vi "Create Test Configuration.vi"() -> (0 "error out":errorcluster, 1 "Channel Names":string[](array[string]), 2 "Lines":T1[](array[typedef]), 3 "Module Configuration":refnum<class "Sequencer Module configuration.lvclass">, 4 "Channels":refnum<class "TBM channel.lvclass">[](array[class]), 5 "instance identifier":string)   [LabVIEW 2015, in "Sequencer Module tests.lvlib"]
doc: "This VI creates a standard test configuration for other unit tests. It currently creates and adds one line with every datatype to the module configuration."
uses:
  Sequencer Module tests.lvlib
  module/configuration/Sequencer Module configuration.lvclass
  <vilib>/NI/Tag Bus Module Framework/channel/TBM channel.lvclass
  module/configuration/Line.ctl
  classes/Sequence/Config/Sequence Config.lvclass
  classes/Result Processor/Config/ResultProcessor Config.lvclass
  classes/Report/On-The-Fly/Config/OnTheFlyReport Config.lvclass
  classes/Report Formatters/csv/Config/csv-formatter Config.lvclass
  <vilib>/NI/Tag Bus/tag/tag descriptor.lvclass/tag descriptor.ctl
  <vilib>/NI/Configuration Framework/serializable configuration/NISE_CEF_serializable configuration.lvclass
  <vilib>/NI/Tag Bus/tag/tag descriptor.lvclass
panel:
  out "Line Names":string[](array[string])
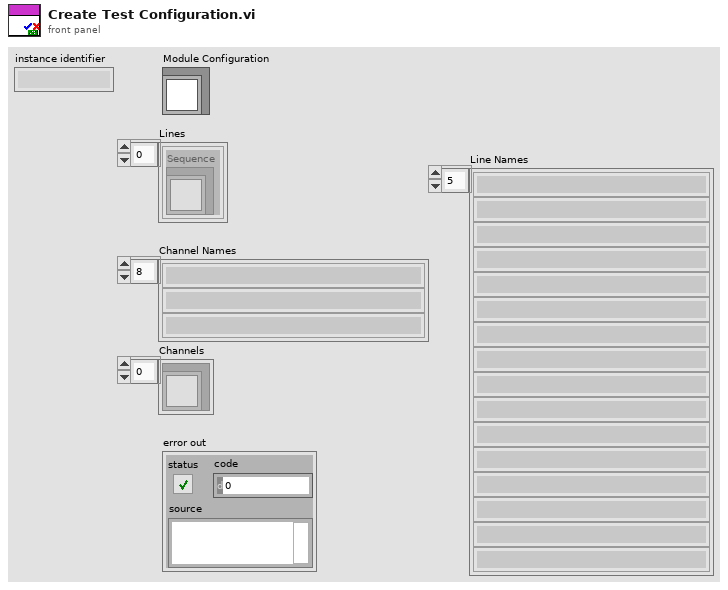
[diagram p1: front panel]
types:
  T1 = typedef "Sequencer Module configuration.lvclass/Line.ctl" = cluster{"Sequence":refnum<class "Sequence Config.lvclass">}
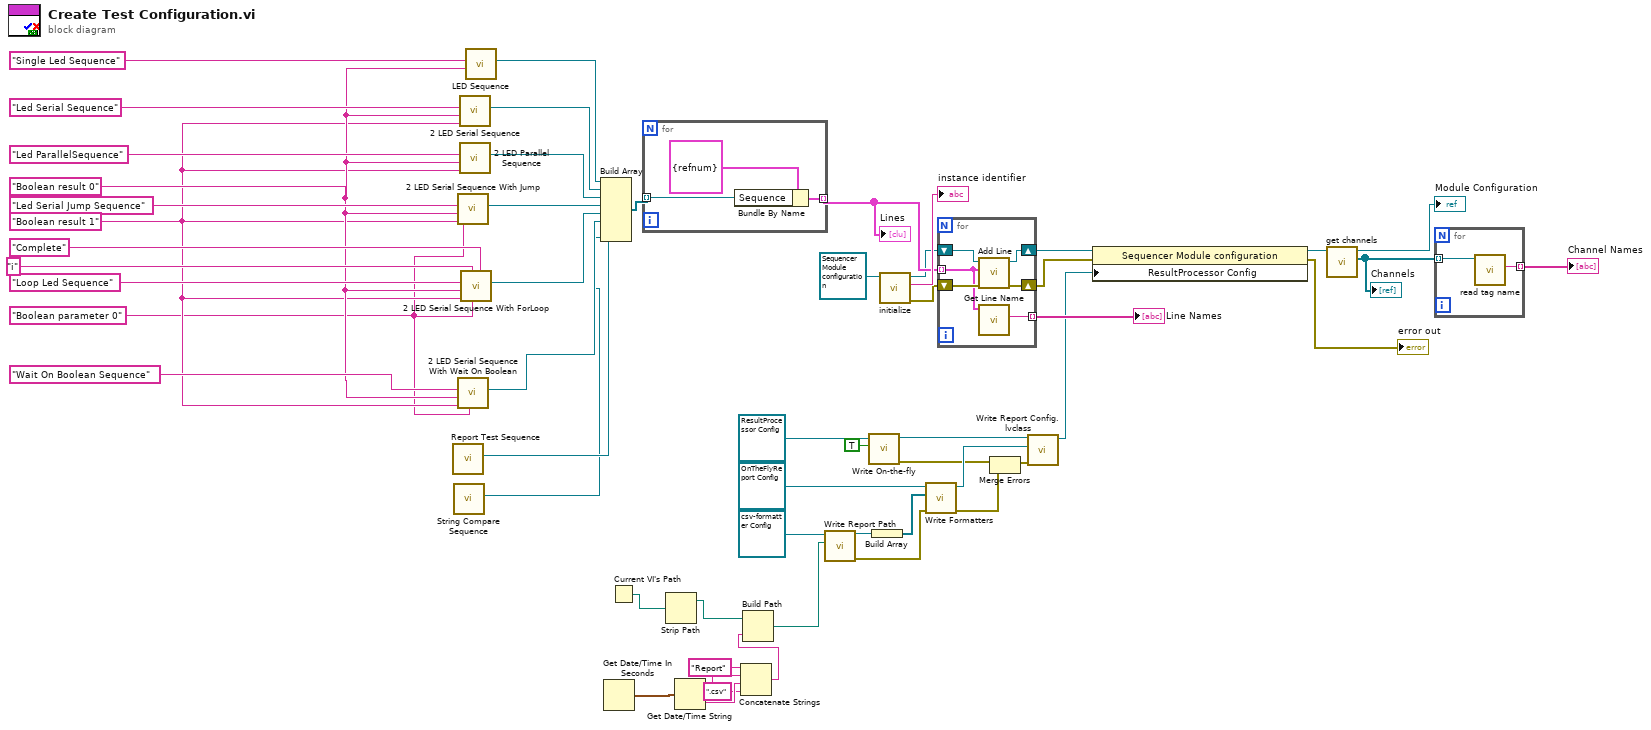
[diagram p0: block diagram]
diagram:
  w30 = "Boolean parameter 0" ("Tag Name")
  w31 = "Boolean result 1" ("Tag Name")
  w32 = "Boolean result 0" ("Tag Name")
  n1 = call "Report Test Sequence.vi"() -> ("Sequence"=w28:refnum<class "Sequence Config.lvclass">)  [unwired: 11 in]
  n2 = call "String Compare Sequence.vi"() -> ("Sequence"=w27:refnum<class "Sequence Config.lvclass">)  [unwired: 11 in]
  n3 = call "2 LED Serial Sequence With Jump.vi"("Jump Tag Name"=w30, "Tag Name 2"=w31, "Tag Name 1"=w32, "Name"="Led Serial Jump Sequence") -> ("Sequence out"=w38:refnum<class "Sequence Config.lvclass">)  [unwired: 7 in]
  n4 = call "2 LED Serial Sequence With Wait On Boolean.vi"("Jump Tag Name"=w30, "Tag Name 2"=w31, "Tag Name 1"=w32, "Name"="Wait On Boolean Sequence") -> ("Sequence out"=w29:refnum<class "Sequence Config.lvclass">)  [unwired: 7 in]
  n5 = call "2 LED Serial Sequence.vi"("Tag Name 2"=w31, "Tag Name 1"=w32, "Name"="Led Serial Sequence") -> ("Sequence out"=w39:refnum<class "Sequence Config.lvclass">)  [unwired: 8 in]
  n6 = call "2 LED Parallel Sequence.vi"("Tag Name 2"=w31, "Tag Name 1"=w32, "Name"="Led ParallelSequence") -> ("Sequence out"=w36:refnum<class "Sequence Config.lvclass">)  [unwired: 8 in]
  n7 = call "2 LED Serial Sequence With ForLoop.vi"("Completed Tag name"="Complete", "Jump Tag Name"=w30, "Iteration Tag Name"="i", "Tag Name 2"=w31, "Tag Name 1"=w32, "Name"="Loop Led Sequence") -> ("Sequence out"=w37:refnum<class "Sequence Config.lvclass">)  [unwired: 5 in]
  n8 = call "LED Sequence.vi"("Tag Name"=w32, "Name"="Single Led Sequence") -> ("Sequence out"=w40:refnum<class "Sequence Config.lvclass">)  [unwired: 9 in]
  n9 = Build Array(w40, w39, w36, w38, w37, w29, w28, w27) -> (w35:refnum<class "Sequence Config.lvclass">[])
  n10 = Get Date/Time In Seconds() -> (seconds since 1Jan1904=w13:timestamp)
  n11 = Current VI's Path() -> (path=w15:path)
  n12 = for {
    tunnel: [w58] -> w53 mode=indexing
    tunnel: w35 -> [w56] mode=indexing
    n13 = Bundle By Name(cluster=T1 {"Sequence"=refnum} ("Line"), "Sequence"=w56) -> (w58:T1)
  }
  "Lines" <- w53
  n14 = Strip Path(path=w15) -> (stripped path=w14:path)  [unwired: 1 out]
  n15 = Get Date/Time String(seconds (now)=w13) -> (date string=w12:string, time string=w11:string)  [unwired: 2 in]
  n16 = Concatenate Strings("Report" ("string"), w12, w11, ".csv" ("string")) -> (w8:string)
  n17 = Build Path(base path=w14, name or relative path=w8) -> (appended path=w7:path)
  n18 = call-dynamic "Write Report Path.vi"("Report Path"=w7, "csv-formatter Config in"=refnum<class "csv-formatter Config.lvclass"> refnum ("csv-formatter Config.lvclass")) -> ("error out"=w6:errorcluster, "csv-formatter Config out"=w16:refnum<class "csv-formatter Config.lvclass">)  [unwired: 8 in]
  n19 = call-dynamic "Write On-the-fly.vi"("On-the-fly?"=TRUE, "ResultProcessor Config in"=refnum<class "ResultProcessor Config.lvclass"> refnum) -> ("error out"=w1:errorcluster, "ResultProcessor Config out"=w4:refnum<class "ResultProcessor Config.lvclass">)  [unwired: 8 in]
  n20 = Build Array(w16) -> (w24:refnum<class "csv-formatter Config.lvclass">[])
  n21 = call <vilib>:"initialize.vi"("configuration in"=refnum<class "Sequencer Module configuration.lvclass"> refnum ("tag bus configurable plugin module configuration")) -> ("error out"=w54:errorcluster, "identifier"=→"instance identifier":string, "configuration out"=w51:refnum<class "Sequencer Module configuration.lvclass">)  [unwired: 8 in]
  n22 = call-dynamic "Write Formatters.vi"("error in (no error)"=w6, "Formatters"=w24, "OnTheFlyReport Config in"=refnum<class "OnTheFlyReport Config.lvclass"> refnum ("OnTheFlyReport Config.lvclass")) -> ("error out"=w23:errorcluster, "OnTheFlyReport Config out"=w25:refnum<class "OnTheFlyReport Config.lvclass">)  [unwired: 7 in]
  n23 = for {
    tunnel: w53 -> [w60] mode=indexing
    shift-right: [w63] -> w22
    shift-left: w51 -> [w64]
    shift-right: [w61] -> w21
    shift-left: w54 -> [w62]
    tunnel: [w59] -> w50 mode=indexing
    n24 = call "Add Line.vi"("error in"=w62, "Line"=w60, "Sequencer Module configuration in"=w64) -> ("error out"=w61:errorcluster, "Sequencer Module configuration out"=w63:refnum<class "Sequencer Module configuration.lvclass">)  [unwired: 6 in, 1 out]
    n25 = call "Get Line Name.vi"("Line in"=w60) -> ("Name"=w59:string)  [unwired: 8 in, 2 out]
  }
  "Line Names" <- w50
  n26 = Merge Errors(w1, w23) -> (w2:errorcluster)
  n27 = call-dynamic "Write Report Config.lvclass.vi"("error in (no error)"=w2, "Report Config.lvclass"=w25, "ResultProcessor Config in"=w4) -> ("ResultProcessor Config out"=w18:refnum<class "ResultProcessor Config.lvclass">)  [unwired: 7 in, 1 out]
  n28 = property class="Sequencer Module configuration"(reference=w22, error in=w21, "ResultProcessor Config"=w18) -> (reference out=w19:refnum<class "Sequencer Module configuration.lvclass">, error out=→"error out":errorcluster)
  n29 = call-dynamic "get channels.vi"("Sequencer Module configuration in"=w19) -> ("channels"=w47:refnum<class "TBM channel.lvclass">[], "Sequencer Module configuration out"=→"Module Configuration":refnum<class "Sequencer Module configuration.lvclass">)  [unwired: 9 in]
  "Channels" <- w47
  n30 = for {
    tunnel: w47 -> [w66] mode=indexing
    tunnel: [w65] -> w49 mode=indexing
    n31 = call <vilib>:"read tag name.vi"("system tag in"=w66) -> ("name"=w65:string)  [unwired: 8 in, 2 out]
  }
  "Channel Names" <- w49
